vi "FPGA Read Array By Name - I8.vi"(8 "error in (no error)":errorcluster, 10 "Indicator":string, 11 "FPGA Session In":refnum<class "FPGA Interface Base.lvclass">) -> (0 "error out":errorcluster, 2 "Array":i8[](array[numeric]), 3 "FPGA Session Out":refnum<class "FPGA Interface Base.lvclass">)   [LabVIEW 2010, in "FPGA Interface Base.lvclass"]
doc: "Reads an entire array of signed 8-bit integer values from a given array indicator or control."
uses:
  <userlib>/_FPGA Interface Advanced Tools/FPGA Interface Base/FPGA Interface Base.lvclass
  <vilib>/rvi/DataTransferAndStorage/Container/Common/niFpgaDataTypeControl.ctl
  <userlib>/_FPGA Interface Advanced Tools/FPGA Interface Base/FPGA Interface Base.lvclass/FPGA Interface Base.ctl
  <vilib>/Utility/error.llb/Error Cluster From Error Code.vi
  <userlib>/_FPGA Interface Advanced Tools/FPGA Interface Base/Accessors/FPGA Read Session.vi
  <userlib>/_FPGA Interface Advanced Tools/FPGA Interface Wrapper/FPGA Interface Wrapper.lvlib
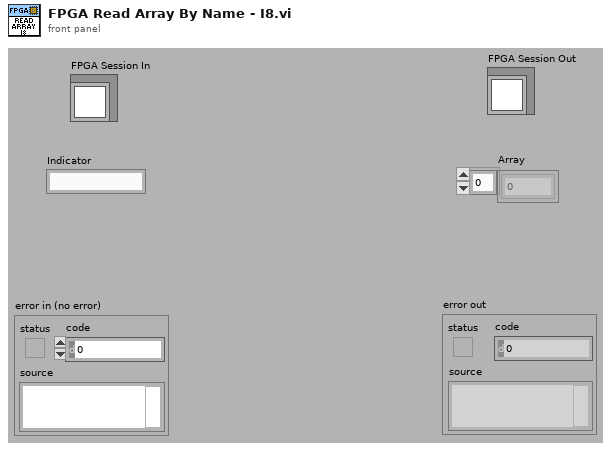
[diagram p1: front panel]
types:
  T1 = typedef "niFpgaDataTypeControl.ctl" = enum32{"Boolean", "I8", "I16", "I32", "I64", "U8", "U16", "U32", "U64", "FXP", "CustomControl"}
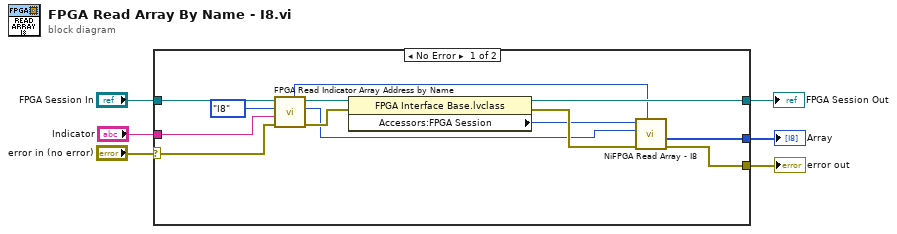
[diagram p0: block diagram]
diagram:
  n1 = case shown="No Error" "error in (no error)" {
    selector: "error in (no error)" -> [w14 w21]
    tunnel: [w15 w21] -> w1
    tunnel: [w16 w20] -> w3
    tunnel: [w19 _] -> w2
    tunnel: "FPGA Session In" -> [w8 w20]
    tunnel: "Indicator" -> [w7 _]
    frame No Error {
      n2 = call <userlib>:"FPGA Read Indicator Array Address by Name.vi"("error in (no error)"=w14, "Name"=w7, "Data Type"=niFpgaDataTypeControl."I8", "FPGA Interface Base in"=w8) -> ("error out"=w13:errorcluster, "Address"=w12:u32, "FPGA Interface Base out"=w11:refnum<class "FPGA Interface Base.lvclass">, "Num Elements"=w9:u32)  [unwired: 3 in, 1 out]
      n3 = property class="FPGA Interface Base.lvclass"(reference=w11, error in=w13) -> (reference out=w16:refnum<class "FPGA Interface Base.lvclass">, error out=w18:errorcluster, "Accessors:FPGA Session"=w17:u32)
      n4 = call <userlib>:"NiFPGA Read Array - I8.vi"("Size"=w9, "error in (no error)"=w18, "Indicator"=w12, "Session"=w17) -> ("error out"=w15:errorcluster, "Array"=w19:i8[])  [unwired: 5 in, 1 out]
    }
    frame Error {
    }
  }
  "error out" <- w1
  "FPGA Session Out" <- w3
  "Array" <- w2
